vi "input data raw.vi"(8 "error in (no error)":errorcluster, 10 "Last row of data file":string[](array[string]), 11 "Automation in":refnum<class "Automation.lvclass">) -> (0 "error out":errorcluster, 3 "Automation out":refnum<class "Automation.lvclass">)   [LabVIEW 2019, in "Automation.lvclass"]
uses:
  Automation.lvclass
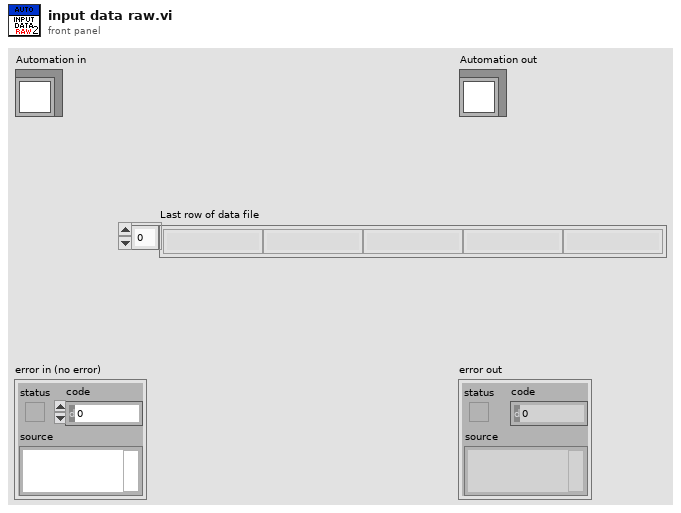
[diagram p1: front panel]
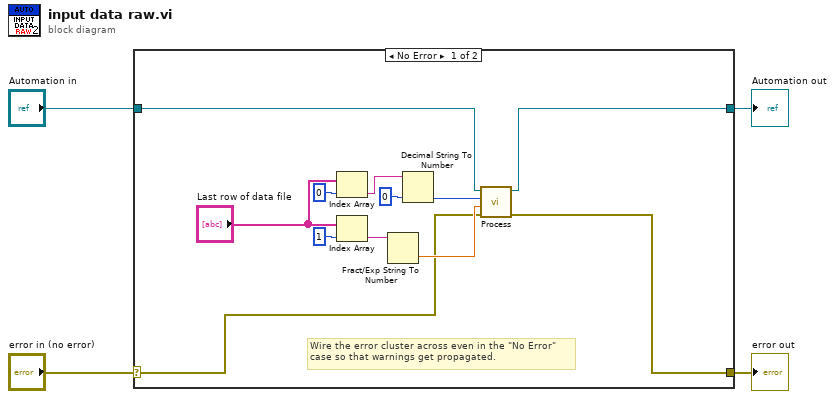
[diagram p0: block diagram]
diagram:
  n1 = case shown="No Error" "error in (no error)" {
    selector: "error in (no error)" -> [w5 w18]
    tunnel: [w6 w18] -> w3
    tunnel: [w7 w17] -> w1
    tunnel: "Automation in" -> [w8 w17]
    frame No Error {
      # "Wire the error cluster across even in the \"No Error\"\ncase so that warnings get propagated."
      n2 = Index Array(array="Last row of data file", index=0) -> (element=w14:string)
      n3 = Index Array(array="Last row of data file", index=1) -> (element=w13:string)
      n4 = Fract/Exp String To Number(string=w13) -> (number=w9:dbl)  [unwired: 3 in, 1 out]
      n5 = Decimal String To Number(string=w14, default (0L)=i64 0 ("default (0 I32)")) -> (number=w10:i64)  [unwired: 1 in, 1 out]
      n6 = call "Process.vi"("error in (no error)"=w5, "New polarization"=w9, "New eventnum"=w10, "Automation in"=w8) -> ("error out"=w6:errorcluster, "Automation out"=w7:refnum<class "Automation.lvclass">)  [unwired: 5 in, 1 out]
    }
    frame Error {
    }
  }
  "error out" <- w3
  "Automation out" <- w1
